vi "audio_play.vi"(6 "Stop":bool, 11 "Bypass":bool) -> ()   [LabVIEW 2013]
uses:
  <vilib>/sound2/lvsound2.llb/Sound Data Format.ctl
  <vilib>/sound2/lvsound2.llb/Sound File Position.ctl
  <vilib>/sound2/lvsound2.llb/Sound File Read Open.vi
  <vilib>/sound2/lvsound2.llb/Sound File Read (DBL).vi
  <vilib>/Analysis/3filter.llb/FIR Filter (DBL).vi
  <vilib>/sound2/lvsound2.llb/Sound Output Write (DBL).vi
  <vilib>/Analysis/NI_AALBase.lvlib
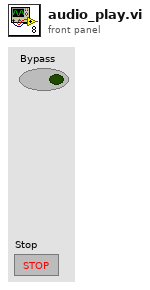
[diagram p1: front panel]
types:
  T1 = typedef "Sound Data Format.ctl" = cluster{"sample rate (S/s)":dbl, "number of channels":i32, "bits per sample":i32}
  T2 = typedef "Sound Output Task ID.ctl" = u32
  T3 = typedef "Sound File Refnum.ctl" = refnum<file>
  T4 = typedef "Sound File Position.ctl" = u16
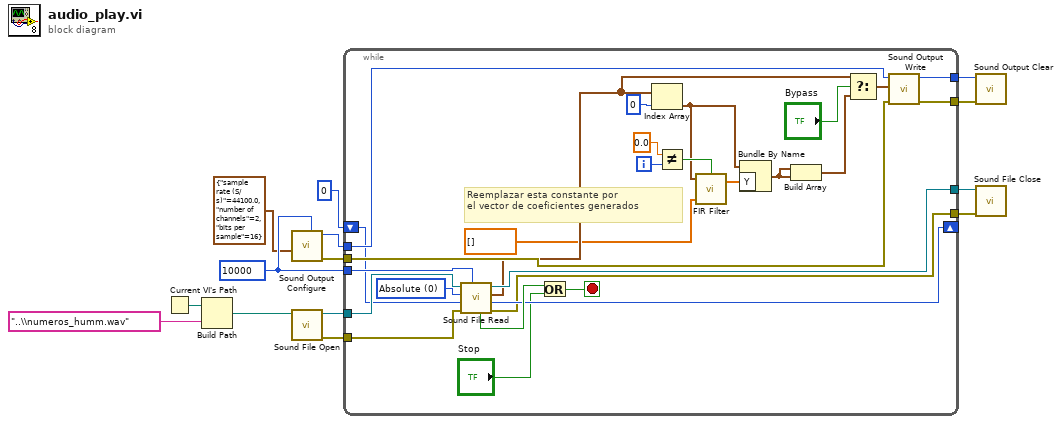
[diagram p0: block diagram]
diagram:
  w11 = 10000 ("number of samples/ch")
  n1 = Current VI's Path() -> (path=w1:path)
  n2 = Build Path(base path=w1, name or relative path="..\\numeros_humm.wav") -> (appended path=w2:path)
  n3 = call <vilib>:"Sound Output Configure.vi"("number of samples/ch"=w11, "sound format"=T1 {"sample rate (S/s)"=44100.0, "number of channels"=2, "bits per sample"=16}) -> ("error out"=w5:errorcluster, "task ID"=w7:T2)  [unwired: 8 in]
  n4 = call-poly <vilib>:"Sound File Open.vi"("path"=w2) -> ("error out"=w12:errorcluster, "sound file refnum"=w9:T3)  [unwired: 9 in]
  n5 = while {
    tunnel: w5 -> [w41]
    tunnel: [w40] -> w6
    tunnel: w7 -> [w39]
    tunnel: [w38] -> w8
    tunnel: w9 -> [w37]
    tunnel: [w36] -> w10
    tunnel: w11 -> [w33]
    shift-right: [w31] -> _
    shift-left: 0 ("offset") -> [w30]
    tunnel: w12 -> [w29]
    tunnel: [w28] -> w13
    i -> [w24]
    stop <- w35 stop-if-true
    w32 = T4 0 items=["Absolute"=0, "Relative"=2] ("position mode")
    # "Reemplazar esta constante por \nel vector de coeficientes generados"
    n6 = call-poly <vilib>:"Sound File Read.vi"("number of samples/ch (-1: all)"=w33, "error in (no error)"=w29, "position offset"=w30, "position mode"=w32, "sound file refnum"=w37) -> ("error out"=w28:errorcluster, "offset"=w31:i32, "data"=w22:waveform(dbl)[], "sound file refnum out"=w36:T3, "end of file?"=w34:bool)  [unwired: 2 in]
    n7 = Or(x=w34, y="Stop") -> (x .or. y?=w35:bool)
    n8 = Index Array(array=w22, index=0) -> (element=w18:waveform(dbl))
    n9 = Not Equal?(x=0.0, y=w24) -> (x != y?=w23:bool)
    n10 = call-poly <vilib>:"FIR Filter.vi"("init/cont (init:F)"=w23, "FIR Coefficients"=dbl[] [], "X"=w18) -> ("Filtered X"=w27:dbl[])  [unwired: 1 in, 1 out]
    n11 = Bundle By Name(cluster=w18, "Y"=w27) -> (w15:waveform(dbl))
    n12 = Build Array(w15, w15) -> (w20:waveform(dbl)[])
    n13 = Select(t=w22, s="Bypass", f=w20) -> (s? t:f=w21:waveform(dbl)[])
    n14 = call-poly <vilib>:"Sound Output Write.vi"("error in (no error)"=w41, "data"=w21, "task ID"=w39) -> ("error out"=w40:errorcluster, "task ID out"=w38:T2)  [unwired: 7 in]
  }
  n15 = call <vilib>:"Sound Output Clear.vi"("error in (no error)"=w6, "task ID"=w8) -> ()  [unwired: 9 in, 1 out]
  n16 = call <vilib>:"Sound File Close.vi"("error in (no error)"=w13, "sound file refnum"=w10) -> ()  [unwired: 9 in, 1 out]
